vi "Get Oscillator Frequency Sweep Step Frequency.vi"(8 "error in (no error)":errorcluster, 11 "VISA resource name":refnum<visa-resource-name>) -> (0 "error out":errorcluster, 1 "Frequency Sweep Type":T1, 2 "Oscillator Frequency Sweep Step":dbl, 3 "VISA resource name out":refnum<visa-resource-name>)   [LabVIEW 2016, in "SR7270 Drivers.lvlib"]
uses:
  SR7270 Drivers.lvlib
  Typedefs/FSTEP--enum.ctl
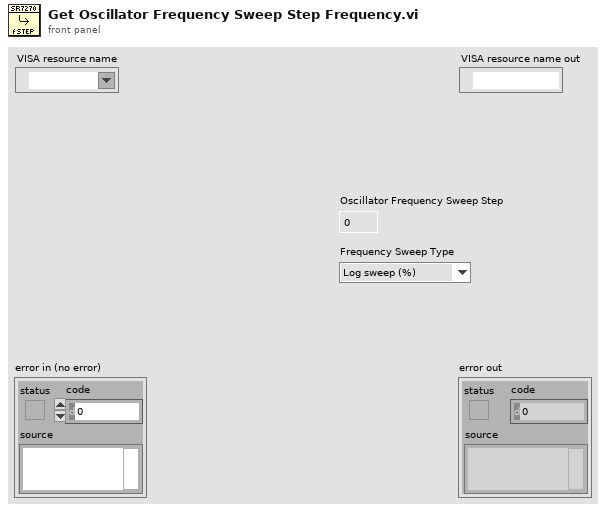
[diagram p1: front panel]
types:
  T1 = typedef "SR7270 Drivers.lvlib/FSTEP--enum.ctl" = enum16{"Log sweep (%)", "Linear sweep (Hz)", "Linear seek sweep (Hz)"}
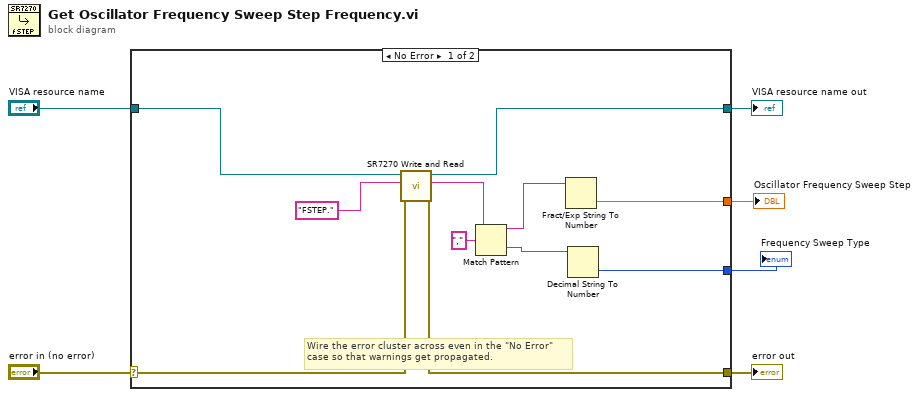
[diagram p0: block diagram]
diagram:
  n1 = case shown="No Error" "error in (no error)" {
    selector: "error in (no error)" -> [w17 w19]
    tunnel: [w16 w19] -> w5
    tunnel: [w7 w18] -> w3
    tunnel: "VISA resource name" -> [w8 w18]
    tunnel: [w14 _] -> w2
    tunnel: [w9 _] -> w1
    frame No Error {
      # "Wire the error cluster across even in the \"No Error\"\ncase so that warnings get propagated."
      n2 = call "SR7270 Write and Read.vi"("error in (no error)"=w17, "Command Name"="FSTEP.", "VISA resource name"=w8) -> ("error out"=w16:errorcluster, "Read"=w12:string, "VISA resource name out"=w7:refnum<visa-resource-name>)  [unwired: 5 in, 1 out]
      n3 = Match Pattern(string=w12, regular expression=",") -> (before substring=w11:string, after substring=w10:string)  [unwired: 1 in, 2 out]
      n4 = Fract/Exp String To Number(string=w11) -> (number=w14:dbl)  [unwired: 3 in, 1 out]
      n5 = Decimal String To Number(string=w10) -> (number=w9:i32)  [unwired: 2 in, 1 out]
    }
    frame Error {
    }
  }
  "error out" <- w5
  "VISA resource name out" <- w3
  "Oscillator Frequency Sweep Step" <- w2
  "Frequency Sweep Type" <- w1
